vi "OPCUA GetPLCModel.vi"(8 "error in (no error)":errorcluster, 11 "Handle":u32) -> (0 "error out":errorcluster, 2 "Model":string, 3 "Handle Out":u32)   [LabVIEW 2018]
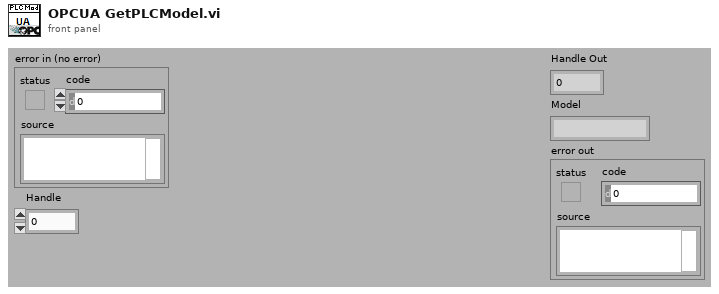
[diagram p1: front panel]
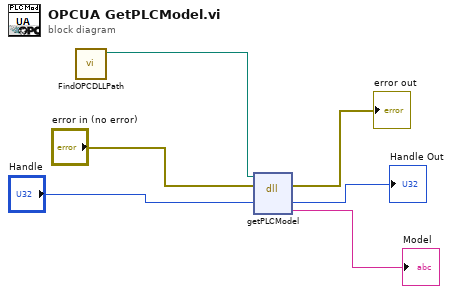
[diagram p0: block diagram]
diagram:
  n1 = call "FindOPCDLLPath.vi"() -> ("DLL Path"=w6:path)  [unwired: 11 in]
  n2 = dll-call lib="D:/src/HUTCDL/Machine/LabWinders/HMI/OPCUA/LVOPCUAInterface.dll" fn="getPLCModel"(path in=w6, error in="error in (no error)", "Handle"="Handle") -> (error out=→"error out":errorcluster, "Handle"=→"Handle Out":u32, "Model"=→"Model":string)  [unwired: 3 in, 1 out]
